vi "Clean gRPC Client.vi"(10 "proto file name":string="data_store_service.proto", 11 "source proto directory":path=path "C:/dev/ASW/Source/Protos") -> (0 "error out":errorcluster)   [LabVIEW 2024, in "gRPC Client Generation.lvlib"]
uses:
  gRPC Client Generation.lvlib
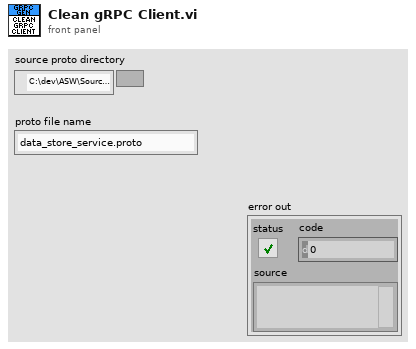
[diagram p1: front panel]
types:
  T1 = typedef "gRPC Client Generation.lvlib/Generation Data.ctl" = cluster{"proto file":path, "imports":path[], "library name":string, "project":path}
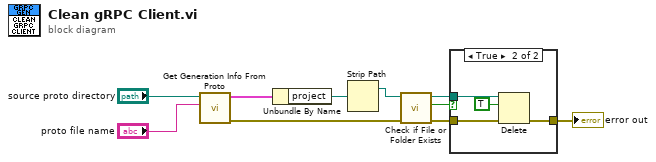
[diagram p0: block diagram]
diagram:
  n1 = call "Get Generation Info From Proto.vi"("proto file name"="proto file name", "source proto directory"="source proto directory") -> ("error out"=w7:errorcluster, "generation data"=w8:T1)  [unwired: 8 in]
  n2 = Unbundle By Name(w8) -> ("project"=w6:path)
  n3 = Strip Path(path=w6) -> (stripped path=w5:path)  [unwired: 1 out]
  n4 = call <vilib>:"Check if File or Folder Exists.vi"("error in (no error)"=w7, "path"=w5) -> ("error out"=w3:errorcluster, "file or folder exists?"=w4:bool, "dup path"=w2:path)  [unwired: 7 in]
  n5 = case shown="True" w4 {
    tunnel: w3 -> [w11 w15]
    tunnel: w2 -> [_ w14]
    tunnel: [w11 w12] -> w1
    frame False {
    }
    frame True {
      n6 = Delete(path (use dialog)=w14, entire hierarchy (F)=TRUE, error in=w15) -> (error out=w12:errorcluster)  [unwired: 2 in, 2 out]
    }
  }
  "error out" <- w1
